vi "Chroma 1905x Series Preset Frequency.vi"(2 "error in":T1, 3 "Frequency":u16(ring) items=["50", "60"], 4 "inst handle in":refnum<visa-resource-name>) -> (0 "error out":T1, 1 "inst handle out":refnum<visa-resource-name>)   [LabVIEW 2025]
uses:
  <instrlib>/Chroma 19052/Chroma 19052.lvlib
panel:
  # "Frequency"
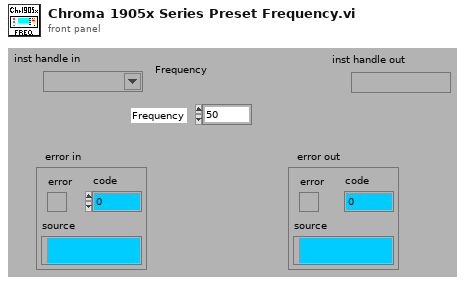
[diagram p1: front panel]
types:
  T1 = cluster{"error":bool, "code":i8, "source":string}
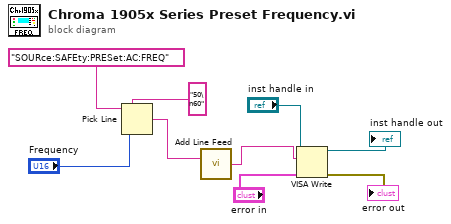
[diagram p0: block diagram]
diagram:
  n1 = Pick Line(string ("")="SOURce:SAFEty:PRESet:AC:FREQ", multi-line string="50\n60", line index="Frequency") -> (output string=w2:string)
  n2 = call <instrlib>:"Add Line Feed.vi"("Cmdstring"=w2) -> ("Concatenated String"=w1:string)
  n3 = VISA Write(VISA resource name="inst handle in", write buffer=w1, error in (no error)="error in") -> (VISA resource name out=→"inst handle out":refnum<visa-resource-name>, error out=→"error out":errorcluster)  [unwired: 1 out]
